vi "Designing.vi"   [LabVIEW 2025]
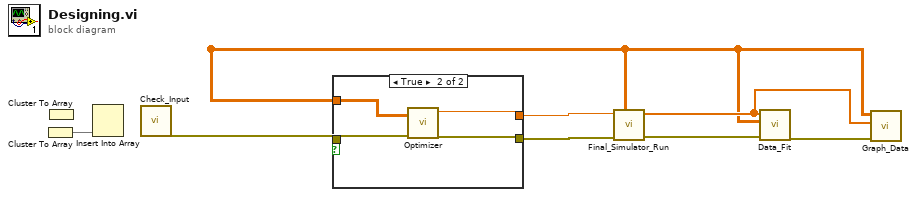
[diagram p0: block diagram]
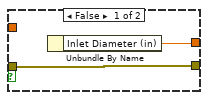
[diagram p2: hidden frame]
diagram:
  n1 = Cluster To Array() -> (array=w11:void[])  [unwired: 1 in]
  n2 = Cluster To Array() -> ()  [unwired: 1 in, 1 out]
  n3 = Insert Into Array(new element=w11) -> ()  [unwired: 2 in, 1 out]
  n4 = call "Check_Input.vi"() -> ("error out"=w12:errorcluster)  [unwired: 11 in]
  n5 = case shown="True" {
    selector: _ -> [_ _]
    tunnel: w12 -> [w18 w22]
    tunnel: [w18 w21] -> w13
    tunnel: [w17 w20] -> w2
    tunnel: [_ w19] -> w1
    frame False {
      n6 = Unbundle By Name() -> ("Inlet Diameter (in)"=w17:dbl)  [unwired: 1 in]
    }
    frame True {
      n7 = call "Optimizer.vi"("Mass Flow (lbm/min) vs. Pressure Drop (inH2O) - Real Data"=w19, "error in"=w22) -> ("error out"=w21:errorcluster, "optimized_diameter"=w20:dbl)  [unwired: 8 in]
    }
  }
  n8 = call "Final_Simulator_Run.vi"("Mass Flow (lbm/min) vs. Pressure Drop (inH2O) - Real Data"=w1, "error in (no error)"=w13, "d_in_guess"=w2) -> ("error out"=w15:errorcluster, "Flow Type"=w5:string, "Flow Type Indicator"=w3:u32, "total_dp_inh2o"=w14:dbl[])  [unwired: 5 in]
  n9 = call "Data_Fit.vi"("error in (no error)"=w15, "Mass Flow (lbm/min) vs. Pressure Drop (inH2O) - Real Data"=w1, "total_dp_inh2o"=w14) -> ("Power - Sim"=w10:string, "Amplitude - Sim"=w9:string, "Power - Empirical"=w8:string, "Amplitude - Empirical"=w7:string, "error out"=w16:errorcluster)  [unwired: 4 in]
  n10 = call "Graph_Data.vi"("error in (no error)"=w16, "total_dp_inh2o"=w14, "Mass Flow (lbm/min) vs. Pressure Drop (inH2O) - Real Data"=w1) -> ("error out"=w6:errorcluster, "Model Validation: Simulated vs. Empirical Airflow Data"=w4:cluster{dbl[], dbl[]}[])  [unwired: 7 in]
